vi "多参手动启动.vi"() -> ()   [LabVIEW 2016]
uses:
  PLC/PLC.lvlib
panel:
  out "仪器状态":T1
  out "步骤流程":T2(ring)
  out "计时":i32
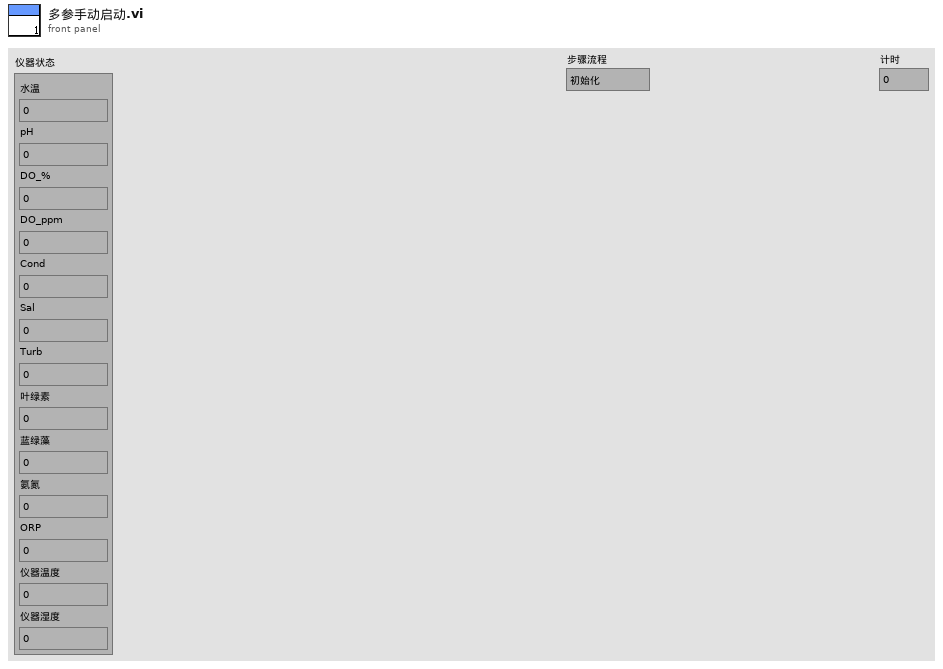
[diagram p1: front panel]
types:
  T1 = cluster{"水温":sgl, "pH":sgl, "DO_%":sgl, "DO_ppm":sgl, "Cond":sgl, "Sal":sgl, "Turb":sgl, "叶绿素":sgl, "蓝绿藻":sgl, "氨氮":sgl, "ORP":sgl, "仪器温度":sgl, "仪器湿度":sgl}
  T2 = enum16{"初始化", "开机", "启动", "读数据", "存数据", "关机", "结束"}
  T3 = cluster{"Y0":bool, "Y1":bool, "Y2":bool, "Y3":bool, "Y4":bool, "Y5":bool, "Y6":bool, "Y7":bool, "Y8":bool, "Y9":bool, "Y10":bool, "Y11":bool, "Y12":bool, "Y13":bool, "Y14":bool, "Y15":bool}
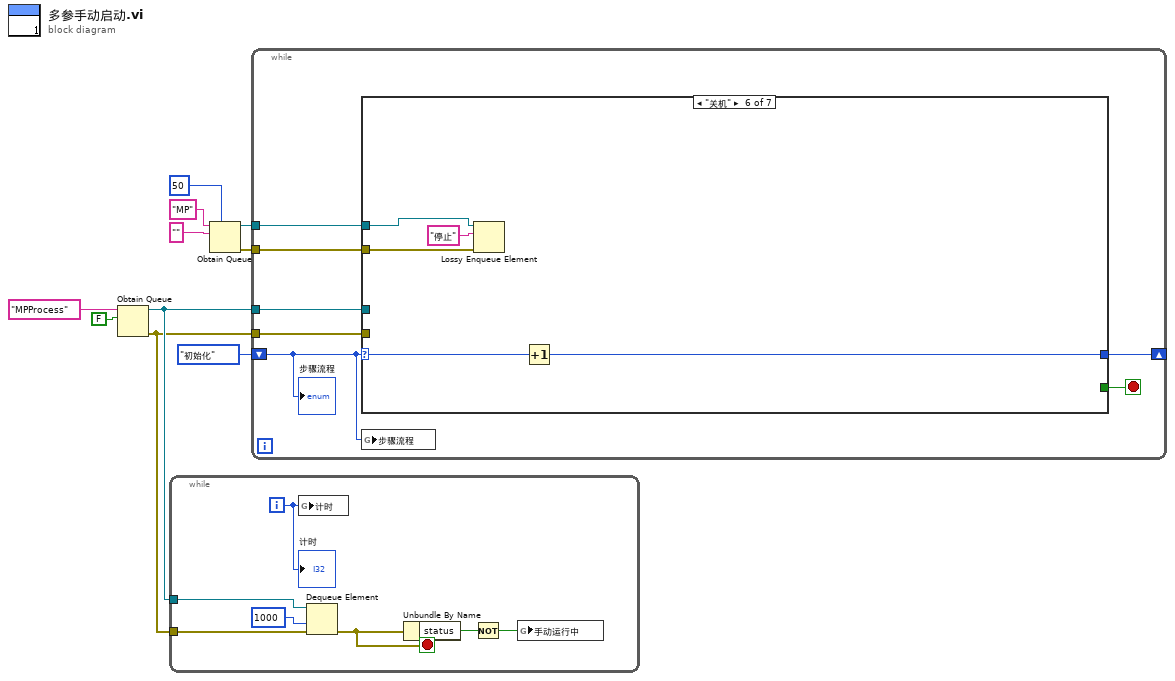
[diagram p0: block diagram]
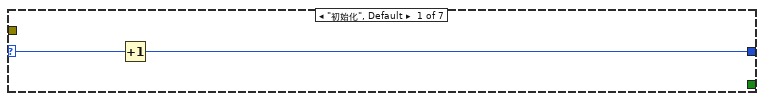
[diagram p2: hidden frame]
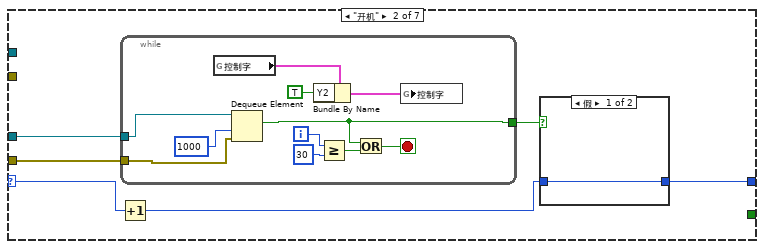
[diagram p3: hidden frame]
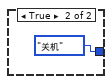
[diagram p4: hidden frame]
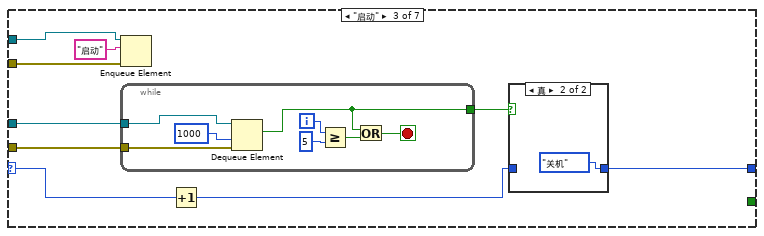
[diagram p5: hidden frame]
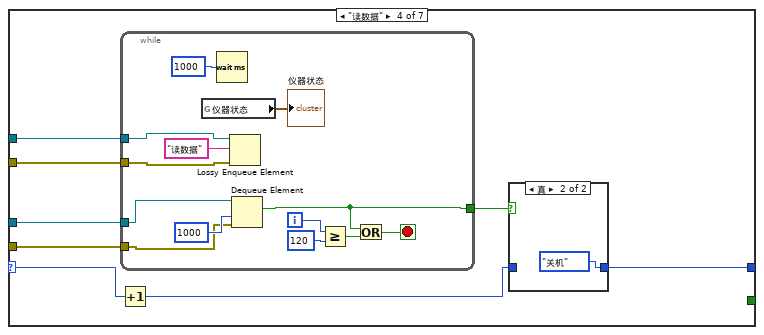
[diagram p7: hidden frame]
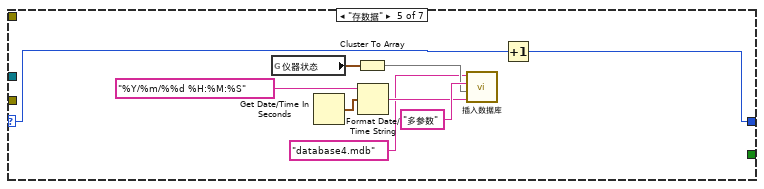
[diagram p9: hidden frame]
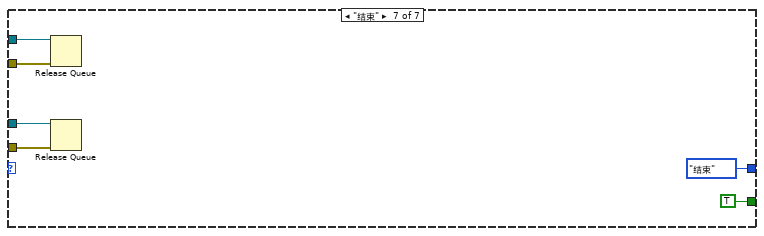
[diagram p10: hidden frame]
diagram:
  n1 = Obtain Queue(name (unnamed)="MPProcess" ("名称（未命名）"), element data type=FALSE) -> (queue out=w3:refnum<queue>, error out=w2:errorcluster)  [unwired: 3 in, 1 out]
  n2 = while {
    tunnel: w3 -> [w17]
    tunnel: w2 -> [w16]
    i -> [w14]
    stop <- w13 stop-if-true
    n3 = global write "多参数全局变量.vi" "计时"(w14) -> ()
    n4 = Dequeue Element(queue=w17, timeout in ms (-1)=1000 ("超时毫秒(-1)"), error in (no error)=w16) -> (error out=w13:errorcluster)  [unwired: 3 out]
    n5 = Unbundle By Name(w13) -> ("status"=w12:bool)
    n6 = Not(x=w12) -> (.not. x?=w11:bool)
    n7 = global write "多参数全局变量.vi" "手动运行中"(w11) -> ()
    "计时" <- w14
  }
  n8 = Obtain Queue(max queue size (-1, unlimited)=50 ("队列最大值（-1，无限）"), name (unnamed)="MP" ("名称（未命名）"), element data type="") -> (queue out=w6:refnum<queue>, error out=w5:errorcluster)  [unwired: 2 in, 1 out]
  n9 = while {
    shift-right: [w23] -> _
    shift-left: T2."初始化" ("枚举") -> [w18]
    tunnel: w6 -> [w22]
    tunnel: w5 -> [w21]
    tunnel: w3 -> [w20]
    tunnel: w2 -> [w19]
    stop <- w24 stop-if-true
    n10 = case shown="\"关机\"" w18 {
      selector: w18 -> [w26 w32 w54 w72 w96 w101 _]
      tunnel: [_ _ _ _ _ _ TRUE] -> w24
      tunnel: [w25 w27 w49 w65 w95 w100 T2."结束" ("枚举")] -> w23
      tunnel: w22 -> [_ _ w46 w71 _ w99 w106]
      tunnel: w21 -> [_ _ w47 w70 _ w98 w105]
      tunnel: w20 -> [_ w31 w53 w69 _ _ w104]
      tunnel: w19 -> [_ w30 w52 w68 _ _ w103]
      frame "初始化", Default {
        n11 = Increment(x=w26) -> (x+1=w25:T2)
      }
      frame "开机" {
        n12 = Increment(x=w32) -> (x+1=w28:T2)
        n13 = while {
          tunnel: w31 -> [w40]
          tunnel: w30 -> [w39]
          tunnel: [w35] -> w29
          i -> [w42]
          stop <- w37 stop-if-true
          n14 = global read "供配电全局变量.vi" "控制字"() -> (w45:T3)
          n15 = Dequeue Element(queue=w40, timeout in ms (-1)=1000 ("超时毫秒(-1)"), error in (no error)=w39) -> (element=w35:bool)  [unwired: 3 out]
          n16 = Bundle By Name(cluster=w45, "Y2"=TRUE) -> (w44:T3)
          n17 = Greater Or Equal?(x=w42, y=30) -> (x >= y?=w36:bool)
          n18 = Or(x=w35, y=w36) -> (x .or. y?=w37:bool)
          n19 = global write "供配电全局变量.vi" "控制字"(w44) -> ()
        }
        n20 = case shown="假" w29 {
          tunnel: w28 -> [w33 _]
          tunnel: [w33 T2."关机"] -> w27
          frame False {
          }
          frame True {
          }
        }
      }
      frame "启动" {
        n21 = Enqueue Element(queue=w46, element="启动" ("元素"), error in (no error)=w47) -> ()  [unwired: 1 in, 3 out]
        n22 = while {
          tunnel: w53 -> [w62]
          tunnel: w52 -> [w61]
          tunnel: [w57] -> w51
          i -> [w64]
          stop <- w58 stop-if-true
          n23 = Dequeue Element(queue=w62, timeout in ms (-1)=1000 ("超时毫秒(-1)"), error in (no error)=w61) -> (element=w57:bool)  [unwired: 3 out]
          n24 = Greater Or Equal?(x=w64, y=5) -> (x >= y?=w59:bool)
          n25 = Or(x=w57, y=w59) -> (x .or. y?=w58:bool)
        }
        n26 = Increment(x=w54) -> (x+1=w50:T2)
        n27 = case shown="真" w51 {
          tunnel: w50 -> [w55 _]
          tunnel: [w55 T2."关机"] -> w49
          frame False {
          }
          frame True {
          }
        }
      }
      frame "读数据" {
        n28 = Increment(x=w72) -> (x+1=w66:T2)
        n29 = while {
          tunnel: w71 -> [w87]
          tunnel: w70 -> [w86]
          tunnel: w69 -> [w81]
          tunnel: w68 -> [w79]
          tunnel: [w76] -> w67
          i -> [w83]
          stop <- w77 stop-if-true
          n30 = global read "多参数全局变量.vi" "仪器状态"() -> (→"仪器状态":T1)
          n31 = Wait (ms)(milliseconds to wait=u32 1000 ("等待时间（毫秒）")) -> ()  [unwired: 1 out]
          n32 = Lossy Enqueue Element(queue=w87, element="读数据" ("元素"), error in (no error)=w86) -> ()  [unwired: 4 out]
          n33 = Dequeue Element(queue=w81, timeout in ms (-1)=1000 ("超时毫秒(-1)"), error in (no error)=w79) -> (element=w76:bool)  [unwired: 3 out]
          n34 = Greater Or Equal?(x=w83, y=120) -> (x >= y?=w78:bool)
          n35 = Or(x=w76, y=w78) -> (x .or. y?=w77:bool)
        }
        n36 = case shown="真" w67 {
          tunnel: w66 -> [w73 _]
          tunnel: [w73 T2."关机"] -> w65
          frame False {
          }
          frame True {
          }
        }
      }
      frame "存数据" {
        n37 = global read "多参数全局变量.vi" "仪器状态"() -> (w88:T1)
        n38 = Get Date/Time In Seconds() -> (seconds since 1Jan1904=w92:timestamp)
        n39 = Cluster To Array(cluster=w88) -> (array=w93:sgl[])
        n40 = Format Date/Time String(time format string (%c)="%Y/%m/%%d %H:%M:%S" ("时间格式字符串(%c)"), seconds (now)=w92) -> (date/time string=w90:string)  [unwired: 1 in]
        n41 = call "插入数据库.vi"("时间戳"=w90, "插入数值"=w93, "table"="多参数", "database"="database4.mdb") -> ()  [unwired: 8 in]
        n42 = Increment(x=w96) -> (x+1=w95:T2)
      }
      frame "关机" {
        n43 = Lossy Enqueue Element(queue=w99, element="停止" ("元素"), error in (no error)=w98) -> ()  [unwired: 4 out]
        n44 = Increment(x=w101) -> (x+1=w100:T2)
      }
      frame "结束" {
        n45 = Release Queue(queue=w106, error in (no error)=w105) -> ()  [unwired: 1 in, 3 out]
        n46 = Release Queue(queue=w104, error in (no error)=w103) -> ()  [unwired: 1 in, 3 out]
      }
    }
    n47 = global write "多参数全局变量.vi" "步骤流程"(w18) -> ()
    "步骤流程" <- w18
  }
